vi "Calculate-temperature-value.vi"(8 "error in":errorcluster, 9 "Temp. params. ref. in":refnum<data-value>, 10 "Buffer element in":T1 {"Temperature characteristics"."Stand. dev. temperature" format="%#.1f"; "Temperature characteristics"."Min. temperature" format="%#.0f"; "Temperature characteristics"."Max. temperature" format="%#.0f"; "Temperature characteristics"."Average temperature" format="%#.0f"}, 11 "Config. params. ref. in":refnum<data-value>) -> (0 "error IO":errorcluster, 1 "Temp. params. ref.":refnum<data-value>, 2 "Buffer element":T1 {"Temperature characteristics"."Stand. dev. temperature" format="%#.1f"; "Temperature characteristics"."Min. temperature" format="%#.0f"; "Temperature characteristics"."Max. temperature" format="%#.0f"; "Temperature characteristics"."Average temperature" format="%#.0f"}, 3 "Config. params. ref.":refnum<data-value>)   [LabVIEW 2013, in "CameraVision.lvlib" / "CV-Temperature.lvclass"]
uses:
  CV-Temperature.lvclass
  Configuration/CV-Configuration.lvclass
  Buffers/Storage-buffer.ctl
  <vilib>/vision/Image Controls.llb/IMAQ Image.ctl
  Temperature-characteristics.ctl
  Analysis/Characteristics-cluster.ctl
  CV-Temperature.lvclass/CV-Temperature.ctl
  Read Temperature value.vi
  Analysis/CV-Analysis.lvclass
  Buffers/CV-Buffers.lvclass
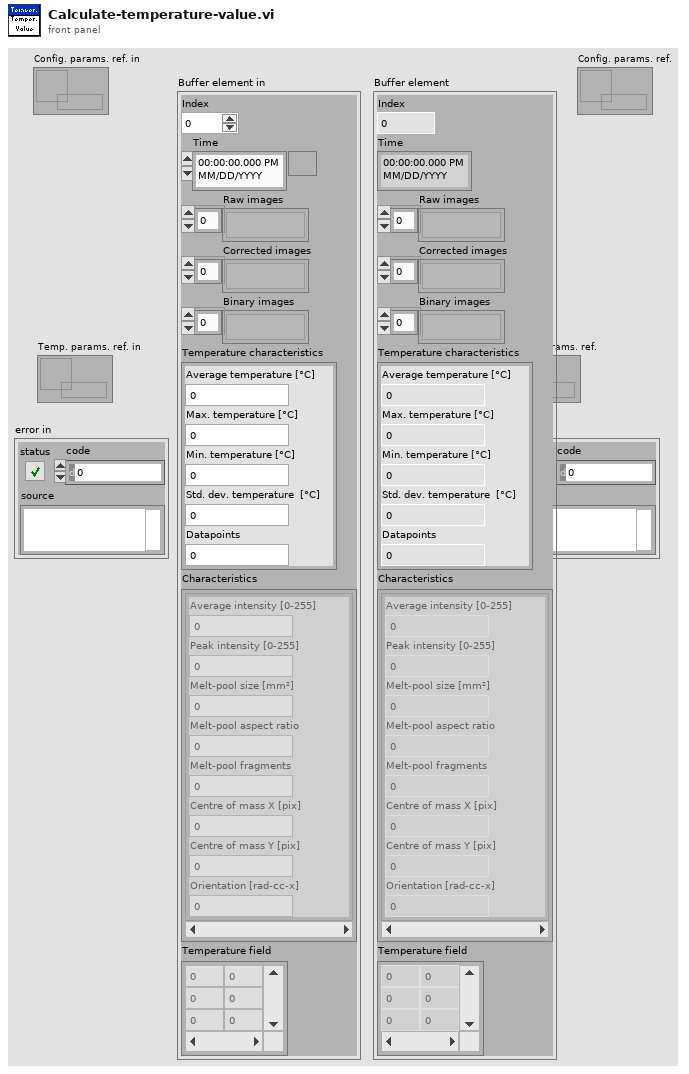
[diagram p1: front panel]
types:
  T1 = typedef "CameraVision.lvlib/CV-Buffers.lvclass/Storage-buffer.ctl" = cluster{"Index":i32, "Time":timestamp, "Raw images":T2[], "Corrected images":T2[], "Binary images":T2[], "Temperature characteristics":T3, "Characteristics":T4[], "Temperature field":dbl[][]}
  T2 = typedef "IMAQ Image.ctl" = refnum<image>
  T3 = typedef "CameraVision.lvlib/CV-Temperature.lvclass/Temperature-characteristics.ctl" = cluster{"Average temperature ":dbl, "Max. temperature":dbl, "Min. temperature":dbl, "Stand. dev. temperature":dbl, "Datapoints":dbl}
  T4 = typedef "CameraVision.lvlib/CV-Analysis.lvclass/Characteristics-cluster.ctl" = cluster{"Average intensity":dbl, "Peak intensity":dbl, "Melt-pool size":dbl, "Melt-pool aspect ratio":dbl, "Melt-pool fragments":dbl, "Centre of mass X":dbl, "Centre of mass Y":dbl, "Orientation":dbl}
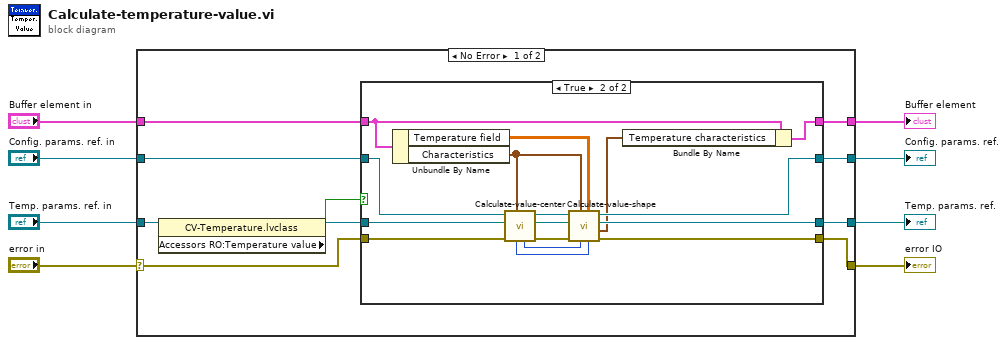
[diagram p0: block diagram]
diagram:
  n1 = case shown="No Error" "error in" {
    selector: "error in" -> [w10 w42]
    tunnel: [w18 w42] -> w7
    tunnel: [w17 w40] -> w2
    tunnel: "Temp. params. ref. in" -> [w16 w41]
    tunnel: "Config. params. ref. in" -> [w13 w40]
    tunnel: [w12 w41] -> w4
    tunnel: "Buffer element in" -> [w11 w39]
    tunnel: [w9 w39] -> w1
    frame No Error {
      n2 = property class="CV-Temperature.lvclass"(reference=w16) -> (reference out=w15:refnum<data-value>, "Accessors RO:Temperature value"=w14:bool)  [unwired: 1 in, 1 out]
      n3 = case shown="True" w14 {
        tunnel: w10 -> [w22 w38]
        tunnel: [w22 w29] -> w18
        tunnel: w15 -> [w21 w33]
        tunnel: [w20 w35] -> w17
        tunnel: w13 -> [w20 w34]
        tunnel: [w21 w30] -> w12
        tunnel: w11 -> [w19 w28]
        tunnel: [w19 w23] -> w9
        frame False {
        }
        frame True {
          n4 = Unbundle By Name(w28) -> ("Temperature field"=w26:dbl[][], "Characteristics"=w25:T4[])
          n5 = call "Calculate-value-center.vi"("Characteristics"=w25, "error in"=w38, "Temp. params. ref. in"=w33, "Config. params. ref. in"=w34) -> ("error IO"=w37:errorcluster, "Temp. params. ref."=w31:refnum<data-value>, "Config. params. ref."=w32:refnum<data-value>, "Center index Y"=w36:i32, "Center index X"=w24:i32)  [unwired: 3 in]
          n6 = call "Calculate-value-shape.vi"("Center index X"=w24, "Temperature field"=w26, "Center index Y"=w36, "Characteristics"=w25, "error in"=w37, "Temp. params. ref. in"=w31, "Config. params. ref. in"=w32) -> ("error IO"=w29:errorcluster, "Temperature characteristics"=w27:T3, "Temp. params. ref. in"=w30:refnum<data-value>, "Config. params. ref."=w35:refnum<data-value>)  [unwired: 1 in]
          n7 = Bundle By Name(cluster=w28, "Temperature characteristics"=w27) -> (w23:T1)
        }
      }
    }
    frame Error {
    }
  }
  "error IO" <- w7
  "Temp. params. ref." <- w4
  "Buffer element" <- w1
  "Config. params. ref." <- w2
